vi "niWLAN - OPPO - 80211abgnGeneration(ref) from waveform.vi"(0 "file path":path, 5 "Without ACK ?":bool, 9 "Idle Time (With Ack)":dbl, 11 "error in":errorcluster) -> (4 "Cluster":T1, 15 "error out":errorcluster)   [LabVIEW 2012]
panel:
  # "Hardware Configuration"
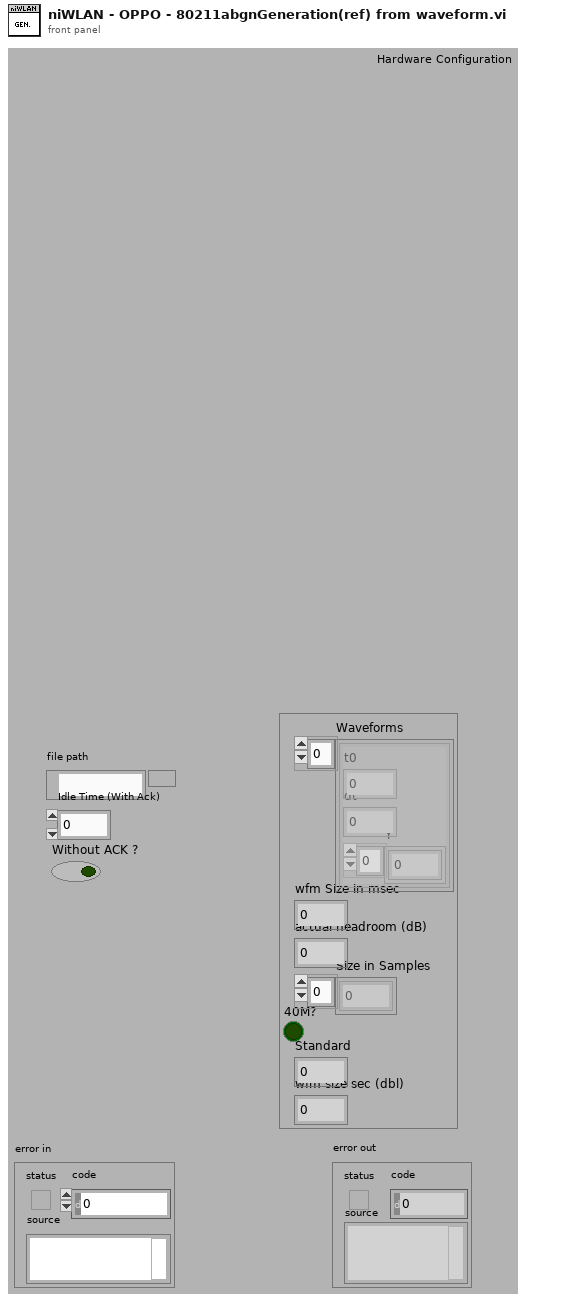
[diagram p1: front panel]
types:
  T1 = cluster{"Waveforms":cluster{"t0":dbl, "dt":dbl, "Y":cdb[]}[], "wfm Size in msec":i32, "actual headroom (dB)":dbl, "Size in Samples":i32[], "40M?":bool, "Standard ":i32, "wfm size sec (dbl)":dbl}
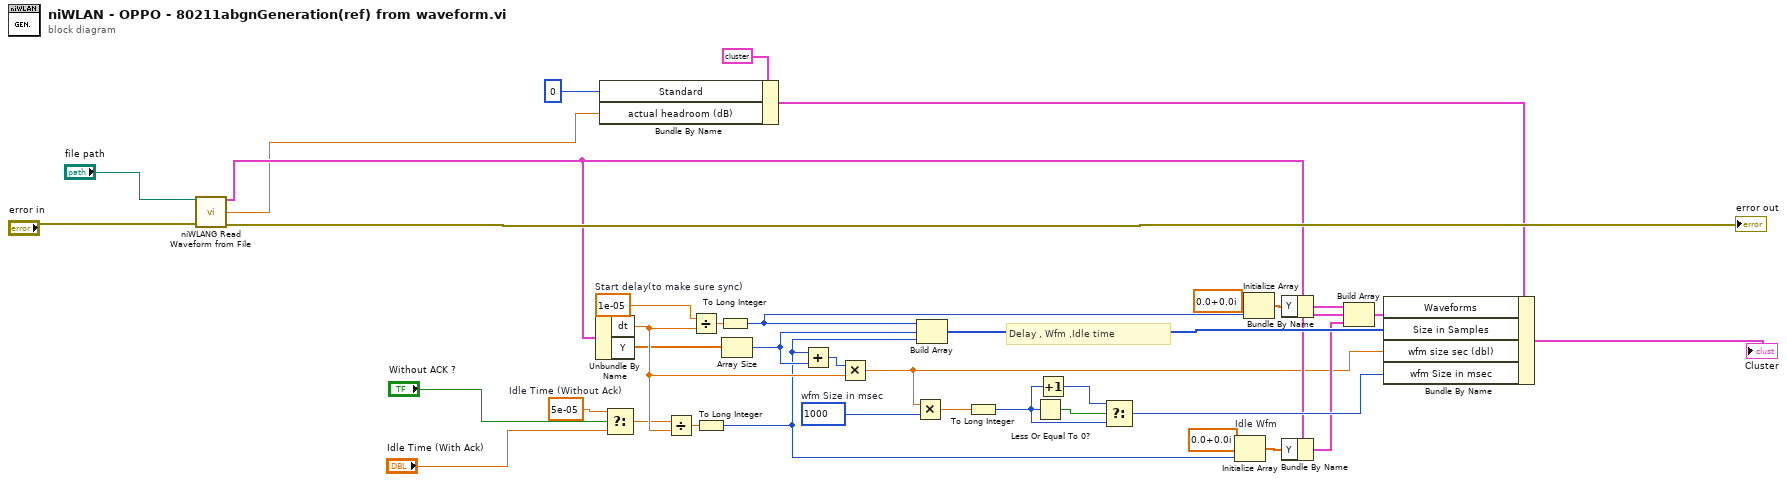
[diagram p0: block diagram]
diagram:
  w16 = 1e-05  # Start delay(to make sure sync)
  w6 = 5e-05  # Idle Time (Without Ack)
  w15 = 1000  # wfm Size in msec
  # "Delay , Wfm ,Idle time"
  n1 = call <vilib>:"niWLANG Read Waveform from File.vi"("file path"="file path", "error in"="error in") -> ("waveform"=w18:cluster{"t0":dbl, "dt":dbl, "Y":cdb[]}, "headroom (dB)"=w8:dbl, "error out"=→"error out":errorcluster)  [unwired: 9 in, 2 out]
  n2 = Unbundle By Name(w18) -> ("dt"=w17:dbl, "Y"=w11:cdb[])
  n3 = Bundle By Name(cluster=T1 {"Waveforms"=[{"t0"=0.0, "dt"=1.25e-08, "Y"=array[800 elements]}, {"t0"=0.0, "dt"=1.25e-08, "Y"=array[85448 elements]}], "wfm Size in msec"=1, "actual headroom (dB)"=0.0, "Size in Samples"=[10000000, 0], "40M?"=TRUE, "Standard "=3, "wfm size sec (dbl)"=0.0} ("Cluster"), "Standard"=0, "actual headroom (dB)"=w8) -> (w9:T1)
  n4 = Select(t=w6, s="Without ACK ?", f="Idle Time (With Ack)") -> (s? t:f=w5:dbl)
  n5 = Divide(x=w5, y=w17) -> (x/y=w20:dbl)
  n6 = Divide(x=w16, y=w17) -> (x/y=w31:dbl)
  n7 = To Long Integer(number=w20) -> (32bit integer=w7:i32)
  n8 = To Long Integer(number=w31) -> (32bit integer=w30:i32)
  n9 = Array Size(array=w11) -> (size(s)=w21:i32)
  n10 = Add(x=w7, y=w21) -> (x+y=w19:i32)
  n11 = Multiply(x=w19, y=w17) -> (x*y=w13:dbl)
  n12 = Multiply(x=w13, y=w15) -> (x*y=w14:dbl)
  n13 = Build Array(w30, w21, w7) -> (w26:i32[])
  n14 = To Long Integer(number=w14) -> (32bit integer=w33:i32)
  n15 = Less Or Equal To 0?(x=w33) -> (x <= 0?=w34:bool)
  n16 = Increment(x=w33) -> (x+1=w32:i32)
  n17 = Select(t=w32, s=w34, f=w33) -> (s? t:f=w25:i32)
  n18 = Initialize Array "Idle Wfm"(cdb 0.0+0.0i ("element"), w7) -> (w23:cdb[])
  n19 = Initialize Array(cdb 0.0+0.0i ("element"), w30) -> (w29:cdb[])
  n20 = Bundle By Name(cluster=w18, "Y"=w29) -> (w28:cluster{"t0":dbl, "dt":dbl, "Y":cdb[]})
  n21 = Bundle By Name(cluster=w18, "Y"=w23) -> (w22:cluster{"t0":dbl, "dt":dbl, "Y":cdb[]})
  n22 = Build Array(w28, w18, w22) -> (w27:cluster{"t0":dbl, "dt":dbl, "Y":cdb[]}[])
  n23 = Bundle By Name(cluster=w9, "Waveforms"=w27, "Size in Samples"=w26, "wfm size sec (dbl)"=w13, "wfm Size in msec"=w25) -> (→"Cluster":T1)
